vi "Write P.vi"(8 "error in (no error)":errorcluster, 10 "P":sgl, 11 "MC Data in":refnum<class "MC Data.lvclass">) -> (0 "error out":errorcluster, 3 "MC Data out":refnum<class "MC Data.lvclass">)   [LabVIEW 2015, in "Alicat Lib.lvlib" / "MC Data.lvclass"]
uses:
  MC Data.lvclass
  MC Data.lvclass/MC Data.ctl
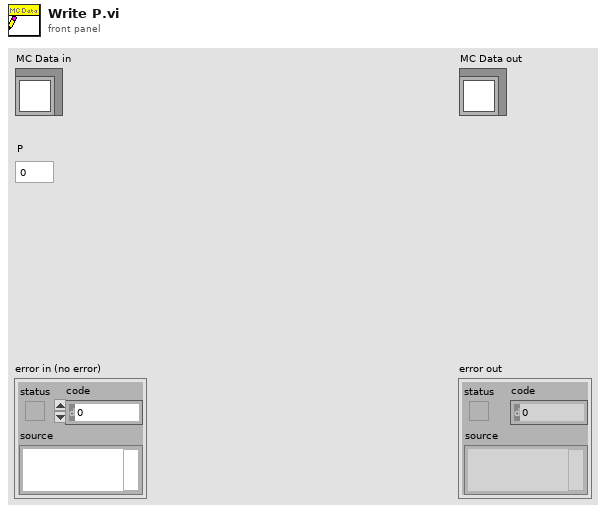
[diagram p1: front panel]
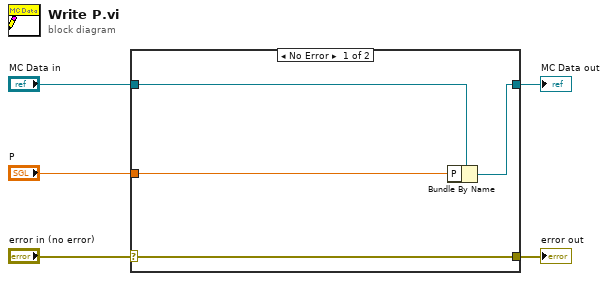
[diagram p0: block diagram]
diagram:
  n1 = case shown="No Error" "error in (no error)" {
    selector: "error in (no error)" -> [w9 w10]
    tunnel: [w9 w10] -> w4
    tunnel: [w7 w11] -> w2
    tunnel: "MC Data in" -> [w8 w11]
    tunnel: "P" -> [w6 _]
    frame No Error {
      n2 = Bundle By Name(cluster=w8, "P"=w6) -> (w7:refnum<class "MC Data.lvclass">)
    }
    frame Error {
    }
  }
  "error out" <- w4
  "MC Data out" <- w2
